vi "Set_Source.vi"(5 "Source Establishment Time (s)":dbl=20.0, 7 "Source Status":T8, 8 "Gas Line Name":T1, 9 "Traverse line":T4 {"Carrier_2 Q (l/min)" format="%#.2f"; "Row Duration (mins)" format="%#.1f"; "Row No" min=0; "Trace Gas Concentration (%)" min=0.0 format="%#_4f"; "Carrier_1 Q (l/min)" format="%#.4f"; "Start X" format="%#.2f"; "Start Y" format="%#.2f"; "Start Z" format="%#.2f"; "End X" format="%#.2f"; "End Y" format="%#.2f"; "End Z" format="%#.2f"; "Tunnel Speed" format="%#.2f"; "Averaging time (mins)" min=0.0 format="%#.2f"}, 10 "Simulate/Run":T7) -> (0 "Status Cluster":T2, 1 "Flowrates (kg/min)":dbl[](array[numeric]) format="%.2f", 2 "Time Source Started":dbl, 3 "Flowrates Achieved?":bool, 4 "Source requested?":bool, 6 "Source Est Time":dbl format="%.2f")   [LabVIEW 2021]
uses:
  ADAM Client/Sub VIs/ADAM Controls/Client_Source_Status.ctl
  Controls/User_Specific_mode.ctl
  Traverse_cluster.ctl
  Spacing.ctl
  Controls/Multi_run_mode.ctl
  Status_Cluster.ctl
  Multi_Run_Status.ctl
  Controls/GMU Gas Line Name.ctl
  ADAM Server/Sub VI's/Gas management/CPP/AalborgServerModes.ctl
  Globals/Extra_Commands_Global.vi
  Globals/Trav_pos_global.vi
  Globals/Preference_global.vi
panel:
  # "X           Y          Z"
  # "Start"
  # "End"
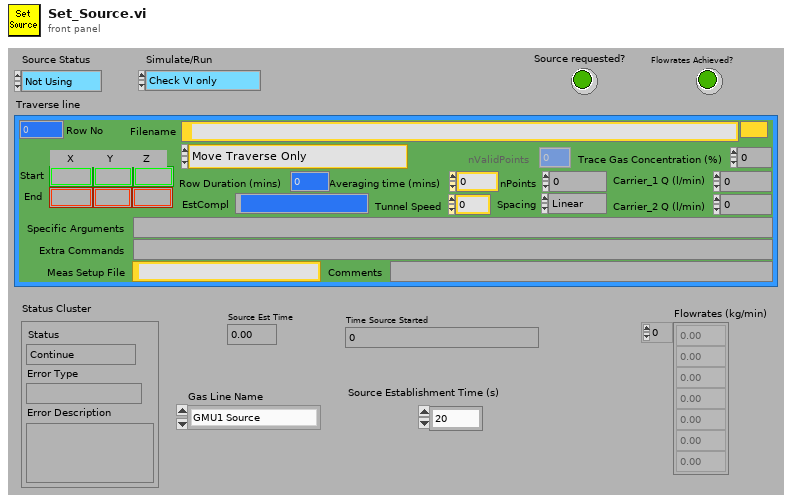
[diagram p1: front panel]
types:
  T1 = typedef "GMU Gas Line Name.ctl" = enum16{"GMU1 Source", "GMU2 Source", "GMU2 Calib", "CPP GRC-A", "CPP GRC-B"}
  T2 = typedef "Status_Cluster.ctl" = cluster{"Status":T3, "Error Type":string, "Error Description":string}
  T3 = typedef "Multi_Run_Status.ctl" = enum16{"Continue", "Continue with Error", "Jump to Next Point", "Jump to Next Row", "Jump To Fall Back", "Terminate Run"}
  T4 = typedef "Traverse_cluster.ctl" = cluster{"Start X":sgl, "Start Y":sgl, "Start Z":sgl, "End X":sgl, "End Y":sgl, "End Z":sgl, "nPoints":i32, "Spacing":T5, "Filename":path, "Tunnel Speed":dbl, "Averaging time (mins)":dbl, "Extra Commands":string, "Carrier_1 Q (l/min)":dbl, "Carrier_2 Q (l/min)":dbl, "Trace Gas Concentration (%)":dbl, "Specific Arguments":string, "Comments":string, "Row No":i32, "Row Type Selector":T6, "EstCompl":string, "Row Duration (mins)":dbl, "nValidPoints":i32, "Meas Setup File":string}
  T5 = typedef "Spacing.ctl" = enum16{"Linear", "Log", "Gauss", "Specified", "N/A"}
  T6 = typedef "Multi_run_mode.ctl" = enum16{"Move Traverse Only", "Set Tunnel Speed Only", "Set Source Only", "Set Measurement Conditions", "Single Measurement", "Vertical Profile", "Lateral Profile", "Longitudinal Profile", "Multi-Axis Profile", "Explore Volume", "Auto Calibrate", "Meas Fast FID Bkgnd", "Check Beam Power", "Scanning Valve Measurement", "Run VI Named:", "Set ADAM Ch", "Wait (minutes)", "Send Message", "Synchronize With:", "Fall Back to this Row", "Turn Off Row Repeating", "Traverse 3D Volume", "Blank Row", "Jump to Fall Back Row"}
  T7 = typedef "User_Specific_mode.ctl" = enum16{"Check VI only", "Run VI"}
  T8 = typedef "Client_Source_Status.ctl" = enum16{"Not Using", "Using", "Must Have"}
  T9 = typedef "AalborgServerModes.ctl" = enum16{"Set Flows", "Check Flows Are Achievable", "Close All MFCs"}
  T10 = cluster{"Carrier_1 Q (l/min)":dbl, "Carrier_2 Q (l/min)":dbl, "Trace Gas Concentration (%)":dbl}
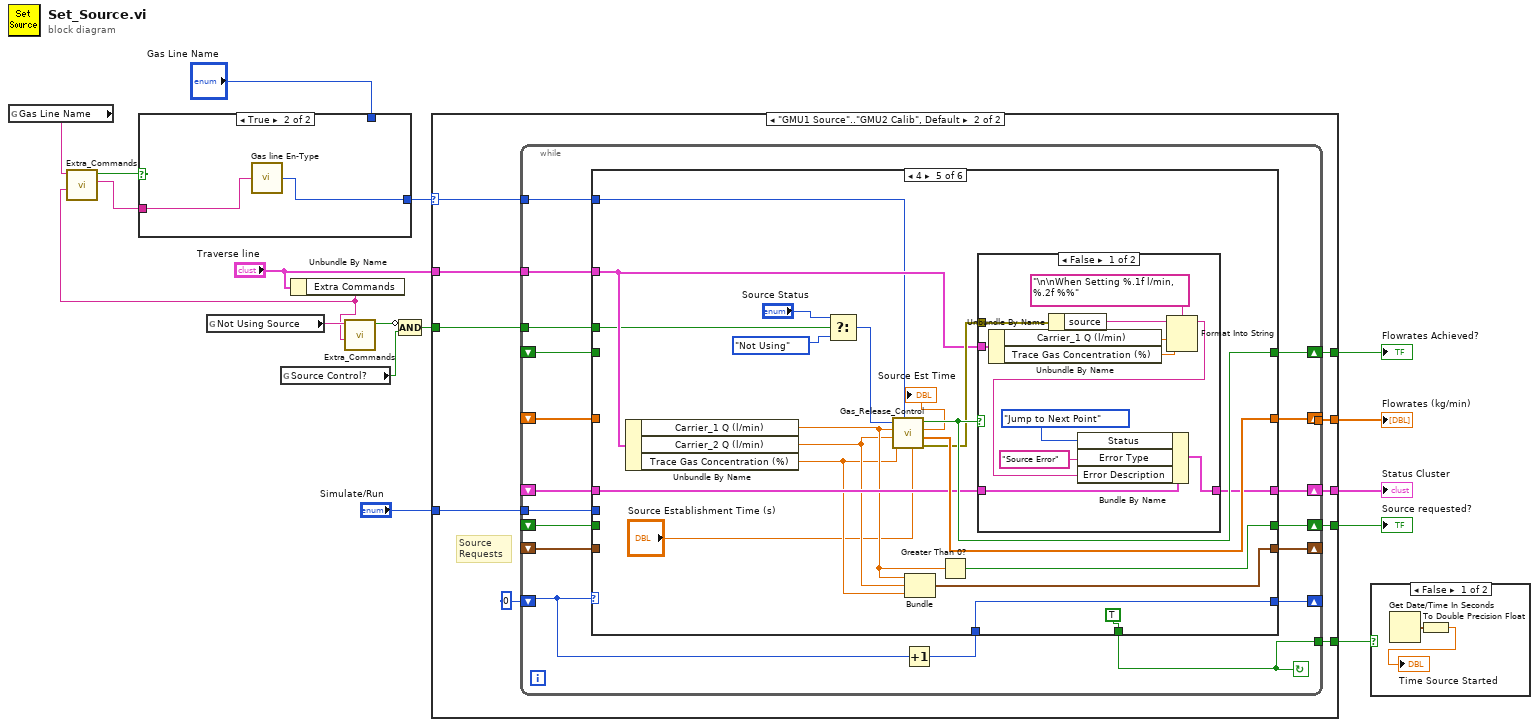
[diagram p0: block diagram]
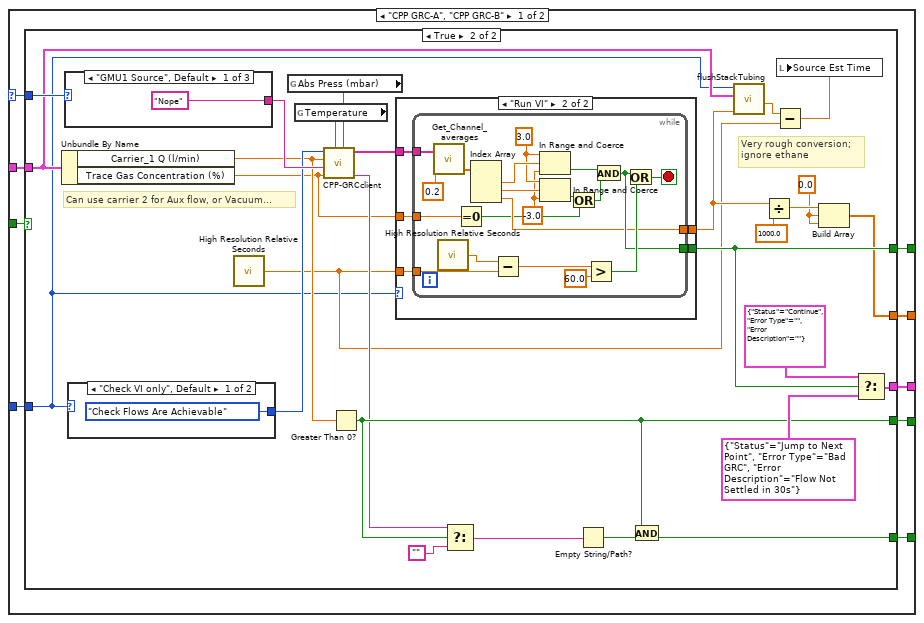
[diagram p3: hidden frame]
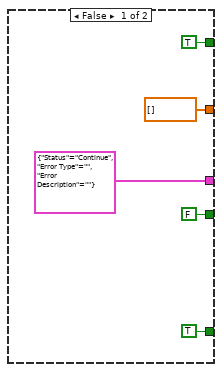
[diagram p4: hidden frame]
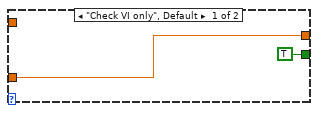
[diagram p5: hidden frame]
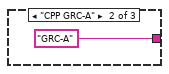
[diagram p6: hidden frame]
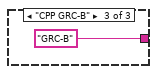
[diagram p7: hidden frame]
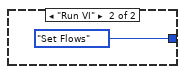
[diagram p8: hidden frame]
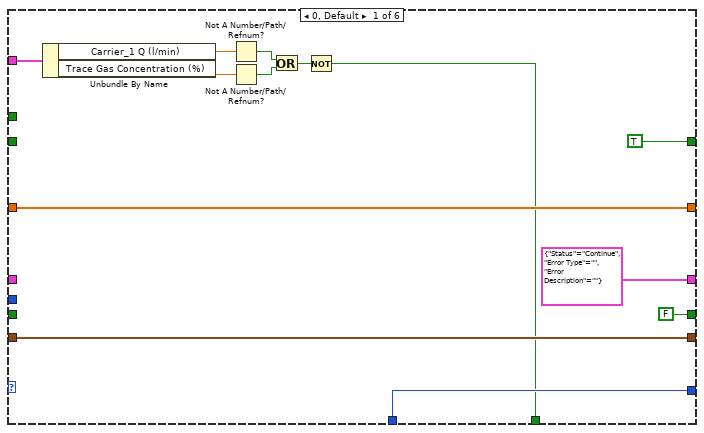
[diagram p9: hidden frame]
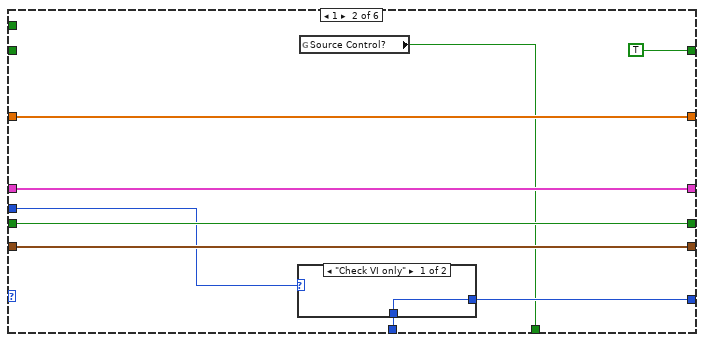
[diagram p10: hidden frame]
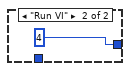
[diagram p11: hidden frame]
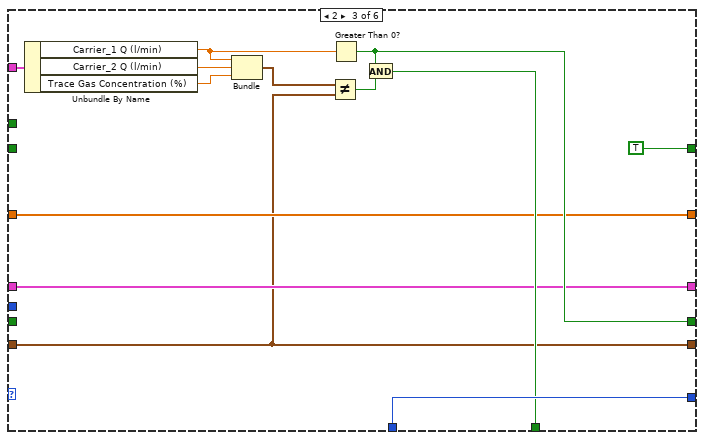
[diagram p12: hidden frame]
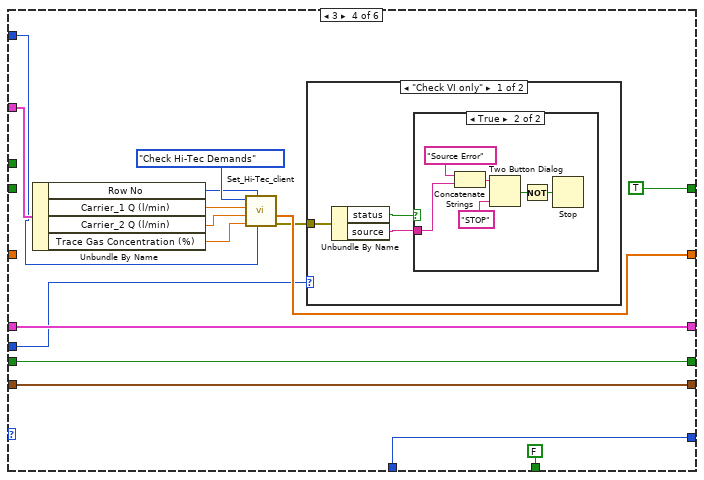
[diagram p13: hidden frame]
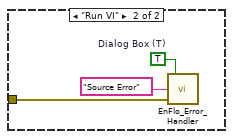
[diagram p15: hidden frame]
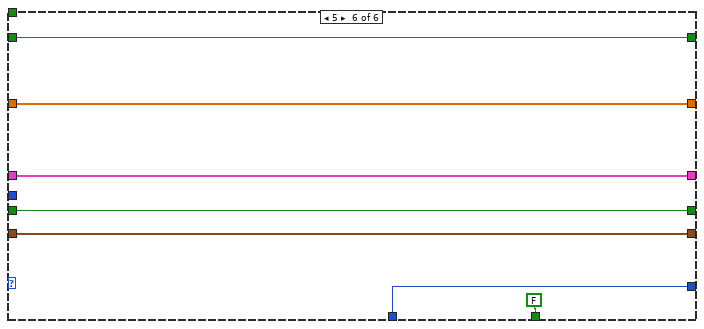
[diagram p17: hidden frame]
diagram:
  n1 = global read "Extra_Commands_Global.vi" "Gas Line Name"() -> (w6:string)
  n2 = global read "Extra_Commands_Global.vi" "Not Using Source"() -> (w10:string)
  n3 = global read "Trav_pos_global.vi" "Source Control?"() -> (w8:bool)
  n4 = Unbundle By Name("Traverse line") -> ("Extra Commands"=w5:string)
  n5 = call "Extra_Commands.vi"("String to Search"=w5, "Command"=w6) -> ("String Value"=w2:string, "Command Found"=w4:bool)  [unwired: 1 in, 3 out]
  n6 = case shown="True" w4 {
    tunnel: [w18 w19] -> w3
    tunnel: w2 -> [_ w20]
    tunnel: "Gas Line Name" -> [w18 _]
    frame False {
    }
    frame True {
      n7 = call "Gas line En-Type.vi"("Gas Line Name String"=w20) -> ("Gas Line Name"=w19:T1)  [unwired: 4 in]
    }
  }
  n8 = call "Extra_Commands.vi"("String to Search"=w5, "Command"=w10) -> ("Command Found"=w7:bool)  [unwired: 1 in, 4 out]
  n9 = Compound Arithmetic op=AND(invert w7, w8) -> (w9:bool)
  n10 = case shown="\"GMU1 Source\"..\"GMU2 Calib\", Default" w3 {
    selector: w3 -> [w24 w96]
    tunnel: [w25 w104] -> w17
    tunnel: [w26 w102] -> w16
    tunnel: [w29 w101] -> w15
    tunnel: [w28 w100] -> w14
    tunnel: "Simulate/Run" -> [w22 w99]
    tunnel: "Traverse line" -> [w23 w98]
    tunnel: [w27 w97] -> w12
    tunnel: w9 -> [w21 w95]
    frame "CPP GRC-A", "CPP GRC-B" {
      n11 = case shown="True" w21 {
        tunnel: [T2 {"Status"=enum."Continue", "Error Type"="", "Error Description"=""} ("Status Cluster") w61] -> w29
        tunnel: [TRUE w58] -> w28
        tunnel: [TRUE w57] -> w27
        tunnel: [FALSE w55] -> w26
        tunnel: [dbl[] [] w52] -> w25
        tunnel: w24 -> [_ w49]
        tunnel: w23 -> [_ w41]
        tunnel: w22 -> [_ w36]
        frame False {
        }
        frame True {
          w51 = 0.0 ("Flowrate (kg/min)")
          # "Very rough conversion;\nignore ethane"
          # "Can use carrier 2 for Aux flow, or Vacuum..."
          n12 = Unbundle By Name(w41) -> ("Carrier_1 Q (l/min)"=w42:dbl, "Trace Gas Concentration (%)"=w35:dbl)
          n13 = case shown="\"GMU1 Source\", Default" w49 {
            tunnel: ["Nope" ("Gas Release System") "GRC-A" ("Gas Release System") "GRC-B" ("Gas Release System")] -> w44
            frame "GMU1 Source", Default {
            }
            frame "CPP GRC-A" {
            }
            frame "CPP GRC-B" {
            }
          }
          n14 = case shown="\"Check VI only\", Default" w36 {
            tunnel: [AalborgServerModes."Check Flows Are Achievable" ("Mode") AalborgServerModes."Set Flows" ("Mode")] -> w43
            frame "Check VI only", Default {
            }
            frame "Run VI" {
            }
          }
          n15 = call <vilib>:"High Resolution Relative Seconds.vi"() -> ("relative seconds"=w38:dbl)
          n16 = global read "Preference_global.vi" "Abs Press (mbar)"() -> (w47:string)
          n17 = global read "Preference_global.vi" "Temperature"() -> (w48:string)
          n18 = call "CPP-GRCclient.vi"("Pressure channel"=w47, "Temperature channel"=w48, "C_dem:(%)"=w35, "Gas Release System"=w44, "Q_dem[Total]:(l/min)"=w42, "Mode"=w43) -> ("errorString"=w45:string, "watchChannels"=w46:string[])  [unwired: 3 in, 1 out]
          n19 = Greater Than 0?(x=w42) -> (x > 0?=w55:bool)
          n20 = case shown="\"Run VI\"" w36 {
            tunnel: [TRUE w69] -> w58
            tunnel: w46 -> [_ w68]
            tunnel: [w64 w67] -> w40
            tunnel: w38 -> [w64 w66]
            tunnel: w35 -> [_ w65]
            frame "Check VI only", Default {
            }
            frame "Run VI" {
              n21 = while {
                tunnel: w68 -> [w89]
                tunnel: w66 -> [w81]
                tunnel: [w75] -> w69
                tunnel: [w74] -> w67
                tunnel: w65 -> [w72]
                stop <- w78 stop-if-true
                w84 = -3.0
                w85 = 3.0
                n22 = call "Get_Channel_averages.vi"("Desired Ch Names"=w89, "Averaging time (mins)"=0.2) -> ("number"=w88:dbl[])  [unwired: 1 in, 2 out]
                n23 = call <vilib>:"High Resolution Relative Seconds.vi"() -> ("relative seconds"=w80:dbl)
                n24 = Equal To 0?(x=w72) -> (x = 0?=w70:bool)
                n25 = Index Array(array=w88) -> (element #1=w87:dbl, element #2=w86:dbl, element #3=w74:dbl)  [unwired: 3 in]
                n26 = Subtract(x=w80, y=w81) -> (x-y=w76:dbl)
                n27 = In Range and Coerce(upper limit=w85, x=w87, lower limit=w84) -> (In Range?=w83:bool)  [unwired: 1 out]
                n28 = In Range and Coerce(upper limit=w85, x=w86, lower limit=w84) -> (In Range?=w82:bool)  [unwired: 1 out]
                n29 = Or(x=w82, y=w70) -> (x .or. y?=w71:bool)
                n30 = Greater?(x=w76, y=60.0) -> (0:w77:bool)
                n31 = And(x=w83, y=w71) -> (x .and. y?=w75:bool)
                n32 = Or(x=w75, y=w77) -> (x .or. y?=w78:bool)
              }
            }
          }
          n33 = Select(t=w45, s=w55, f="") -> (s? t:f=w56:string)
          n34 = Empty String/Path?(string/path=w56) -> (empty?=w62:bool)
          n35 = And(x=w55, y=w62) -> (x .and. y?=w57:bool)
          n36 = call "flushStackTubing.vi"("measQ"=w40, "Traverse line"=w41, "Simulate/Run"=w36) -> ("endTime"=w39:dbl)  [unwired: 8 in]
          n37 = Divide(x=w40, y=1000.0) -> (x/y=w53:dbl)
          n38 = Subtract(x=w39, y=w38) -> (x-y=w37:dbl)
          n39 = local write "Source Est Time"(w37) -> ()
          n40 = Build Array(w53, w51, w51) -> (w52:dbl[])
          n41 = Select(t=T2 {"Status"=enum."Continue", "Error Type"="", "Error Description"=""} ("Status Cluster"), s=w58, f=T2 {"Status"=enum."Jump to Next Point", "Error Type"="Bad GRC", "Error Description"="Flow Not Settled in 30s"} ("Status Cluster")) -> (s? t:f=w61:T2)
        }
      }
    }
    frame "GMU1 Source".."GMU2 Calib", Default {
      # "Source Requests"
      n42 = while {
        shift-left: _ -> [w110]
        shift-right: [w111] -> w100
        shift-left: _ -> [w112]
        shift-right: [w113] -> w101
        shift-left: _ -> [w114]
        shift-right: [w117] -> w102
        shift-left: 0 -> [w116]
        shift-right: [w118] -> _
        shift-left: _ -> [w119]
        shift-right: [w120] -> _
        tunnel: [w120] -> w104
        shift-left: _ -> [w122]
        shift-right: [w121] -> _
        tunnel: w99 -> [w109]
        tunnel: w98 -> [w108]
        tunnel: [w107] -> w97
        tunnel: w96 -> [w106]
        tunnel: w95 -> [w105]
        stop <- w107 continue-if-true
        n43 = Increment(x=w116) -> (x+1=w115:i32)
        n44 = case shown="4" w116 {
          tunnel: [w133 w144 w150 w170 w203 w221] -> w120
          tunnel: w122 -> [w130 w142 w148 w167 _ w225]
          tunnel: [w130 w142 w148 w167 w195 w225] -> w121
          tunnel: w119 -> [w133 w144 w150 _ _ w221]
          tunnel: [FALSE w138 w159 w168 w207 w226] -> w117
          tunnel: [TRUE ("Flowrates Achieved?") TRUE ("Flowrates Achieved?") TRUE ("Flowrates Achieved?") TRUE ("Flowrates Achieved?") w204 w220] -> w111
          tunnel: [w123 w136 w153 FALSE TRUE FALSE] -> w107
          tunnel: [w129 w141 w154 w166 w201 w224] -> w118
          tunnel: w115 -> [w129 w139 w154 w166 w201 w224]
          tunnel: w114 -> [_ w138 _ w168 _ w226]
          tunnel: [T2 {"Status"=enum."Continue", "Error Type"="", "Error Description"=""} ("Status Cluster") w140 w149 w164 w202 w222] -> w113
          tunnel: w112 -> [_ w140 w149 w164 w199 w222]
          tunnel: w110 -> [_ _ _ _ _ w220]
          tunnel: w109 -> [_ w137 _ w162 _ _]
          tunnel: w108 -> [w127 _ w147 w161 w193 _]
          tunnel: w106 -> [_ _ _ w160 w192 _]
          tunnel: w105 -> [_ _ _ _ w191 _]
          frame 0, Default {
            n45 = Unbundle By Name(w127) -> ("Carrier_1 Q (l/min)"=w135:dbl, "Trace Gas Concentration (%)"=w128:dbl)
            n46 = Not A Number/Path/Refnum?(number/path/refnum=w135) -> (NaN/Path/Refnum?=w125:bool)
            n47 = Not A Number/Path/Refnum?(number/path/refnum=w128) -> (NaN/Path/Refnum?=w126:bool)
            n48 = Or(x=w125, y=w126) -> (x .or. y?=w124:bool)
            n49 = Not(x=w124) -> (.not. x?=w123:bool)
          }
          frame 1 {
            n50 = case shown="\"Check VI only\"" w137 {
              tunnel: [w145 4] -> w141
              tunnel: w139 -> [w145 _]
              frame "Check VI only" {
              }
              frame "Run VI" {
              }
            }
            n51 = global read "Trav_pos_global.vi" "Source Control?"() -> (w136:bool)
          }
          frame 2 {
            n52 = Unbundle By Name(w147) -> ("Carrier_1 Q (l/min)"=w156:dbl, "Carrier_2 Q (l/min)"=w158:dbl, "Trace Gas Concentration (%)"=w157:dbl)
            n53 = Bundle("Carrier_1 Q (l/min)"=w156, "Carrier_2 Q (l/min)"=w158, "Trace Gas Concentration (%)"=w157) -> (w152:T10)  [unwired: 1 out]
            n54 = Not Equal?(x=w152, y=w148) -> (x != y?=w155:bool)
            n55 = Greater Than 0?(x=w156) -> (x > 0?=w159:bool)
            n56 = And(x=w159, y=w155) -> (x .and. y?=w153:bool)
          }
          frame 3 {
            n57 = Unbundle By Name(w161) -> ("Row No"=w171:i32, "Carrier_1 Q (l/min)"=w174:dbl, "Carrier_2 Q (l/min)"=w173:dbl, "Trace Gas Concentration (%)"=w172:dbl)
            n58 = call "Set_Hi-Tec_client.vi"("Gas Line Name"=w160, "Row No"=w171, "Strength (% by volume)"=w172, "Carrier_2 Q (l/min)"=w173, "Carrier_1 Q (l/min)"=w174, "Mode"=enum16{"Control Hi-Tec", "Check Hi-Tec Demands"}."Check Hi-Tec Demands") -> ("error out"=w163:errorcluster, "Flowrates (kg/min)"=w170:dbl[])  [unwired: 2 out]
            n59 = case shown="\"Check VI only\"" w162 {
              tunnel: w163 -> [w178 w187]
              frame "Check VI only" {
                n60 = Unbundle By Name(w178) -> ("status"=w176:bool, "source"=w177:string)
                n61 = case shown="True" w176 {
                  tunnel: w177 -> [_ w183]
                  frame False {
                  }
                  frame True {
                    n62 = Concatenate Strings("Source Error" ("Error Type"), w183) -> (w182:string)
                    n63 = Two Button Dialog(message=w182, 1:"STOP" ("F button name (\"Cancel\")")) -> (T button?=w180:bool)  [unwired: 1 out]
                    n64 = Not(x=w180) -> (.not. x?=w179:bool)
                    n65 = Stop(stop? (T)=w179) -> ()
                  }
                }
              }
              frame "Run VI" {
                w185 = TRUE  # Dialog Box (T)
                n66 = call "EnFlo_Error_Handler.vi"("error in (no error)"=w187, "Error Type"="Source Error", "Dialog Box (F)"=w185) -> ()  [unwired: 3 out]
              }
            }
          }
          frame 4 {
            n67 = Unbundle By Name(w193) -> ("Carrier_1 Q (l/min)"=w198:dbl, "Carrier_2 Q (l/min)"=w197:dbl, "Trace Gas Concentration (%)"=w196:dbl)
            n68 = Select(t="Source Status", s=w191, f=Client_Source_Status."Not Using" ("Source Status")) -> (s? t:f=w205:T8)
            n69 = call "Gas_Release_Control.vi"("Source Establishment Time (s)"="Source Establishment Time (s)", "Gas Line Name"=w192, "Strength (% by volume)"=w196, "Carrier_2 Q (l/min)"=w197, "Carrier_1 Q (l/min)"=w198, "Source Status"=w205) -> ("error out"=w194:errorcluster, "Flowrates (kg/min)"=w203:dbl[], "Source Est Time (s)"=→"Source Est Time":dbl, "Flowrates Achieved?"=w204:bool)
            n70 = Bundle("Carrier_1 Q (l/min)"=w198, "Carrier_2 Q (l/min)"=w197, "Trace Gas Concentration (%)"=w196) -> (w195:T10)  [unwired: 1 out]
            n71 = Greater Than 0?(x=w198) -> (x > 0?=w207:bool)
            n72 = case shown="False" w204 {
              tunnel: [w214 w219] -> w202
              tunnel: w199 -> [w215 w219]
              tunnel: w193 -> [w210 _]
              tunnel: w194 -> [w209 _]
              frame False {
                n73 = Unbundle By Name(w210) -> ("Carrier_1 Q (l/min)"=w217:dbl, "Trace Gas Concentration (%)"=w216:dbl)
                n74 = Unbundle By Name(w209) -> ("source"=w208:string)
                n75 = Format Into String(format string="\n\nWhen Setting %.1f l/min, %.2f %%" ("Format String"), initial string=w208, w217, w216) -> (resulting string=w211:string)  [unwired: 1 in, 1 out]
                n76 = Bundle By Name(cluster=w215, "Status"=Multi_Run_Status."Jump to Next Point", "Error Type"="Source Error" ("Bundle Element"), "Error Description"=w211) -> (w214:T2)
              }
              frame True {
              }
            }
          }
          frame 5 {
          }
        }
      }
    }
  }
  "Flowrates (kg/min)" <- w17
  "Source requested?" <- w16
  "Flowrates Achieved?" <- w14
  "Status Cluster" <- w15
  n77 = case shown="False" w12 {
    frame False {
      n78 = Get Date/Time In Seconds() -> (seconds since 1Jan1904=w228:timestamp)
      n79 = To Double Precision Float(number=w228) -> (double precision float=→"Time Source Started":dbl)
    }
    frame True {
    }
  }
